vi "am_modul.vi"() -> ()   [LabVIEW 2015]
uses:
  <vilib>/express/express shared/transition.llb/Dynamic To Waveform Array.vi
  <vilib>/express/express arith-compare/Formula/Block/exnFormulaBlock how many pts in the wave.vi
  <vilib>/express/express shared/ex_Modify Signal Name.vi
  <vilib>/express/express shared/transition.llb/Waveform Array To Dynamic.vi
  <vilib>/express/express arith-compare/Formula/XNode/ExpressFormulaBlockNode.xnode
panel:
  out "String":string
  out "error out":errorcluster
  in  "stop":bool
  out "Graph demod AM-signal":dynamicdata(graph)
  out "f_demod_Hz":u32
  out "K_mod":dbl
  out "Graph AM-signal":dynamicdata(graph)
  in  "A_carry_V":dbl(knob) scale=0.1..0.3
  in  "F_mod_Hz":u32(knob) scale=40.0..280.0
  in  "A_mod_V":dbl(knob) scale=0.0..0.28
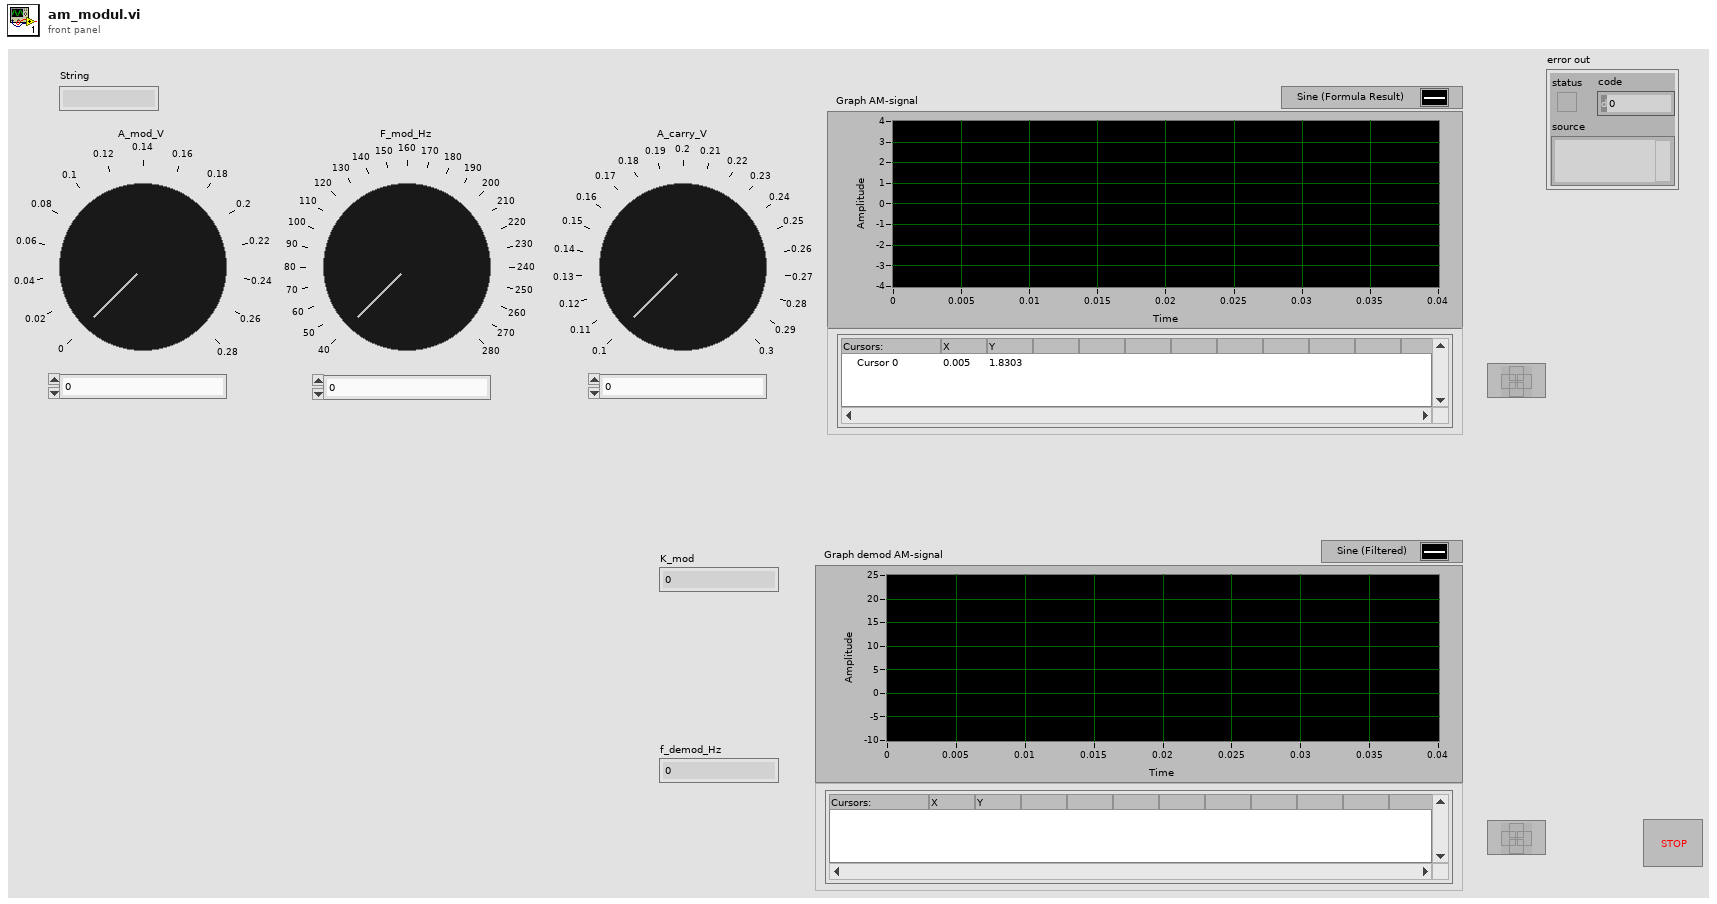
[diagram p1: front panel]
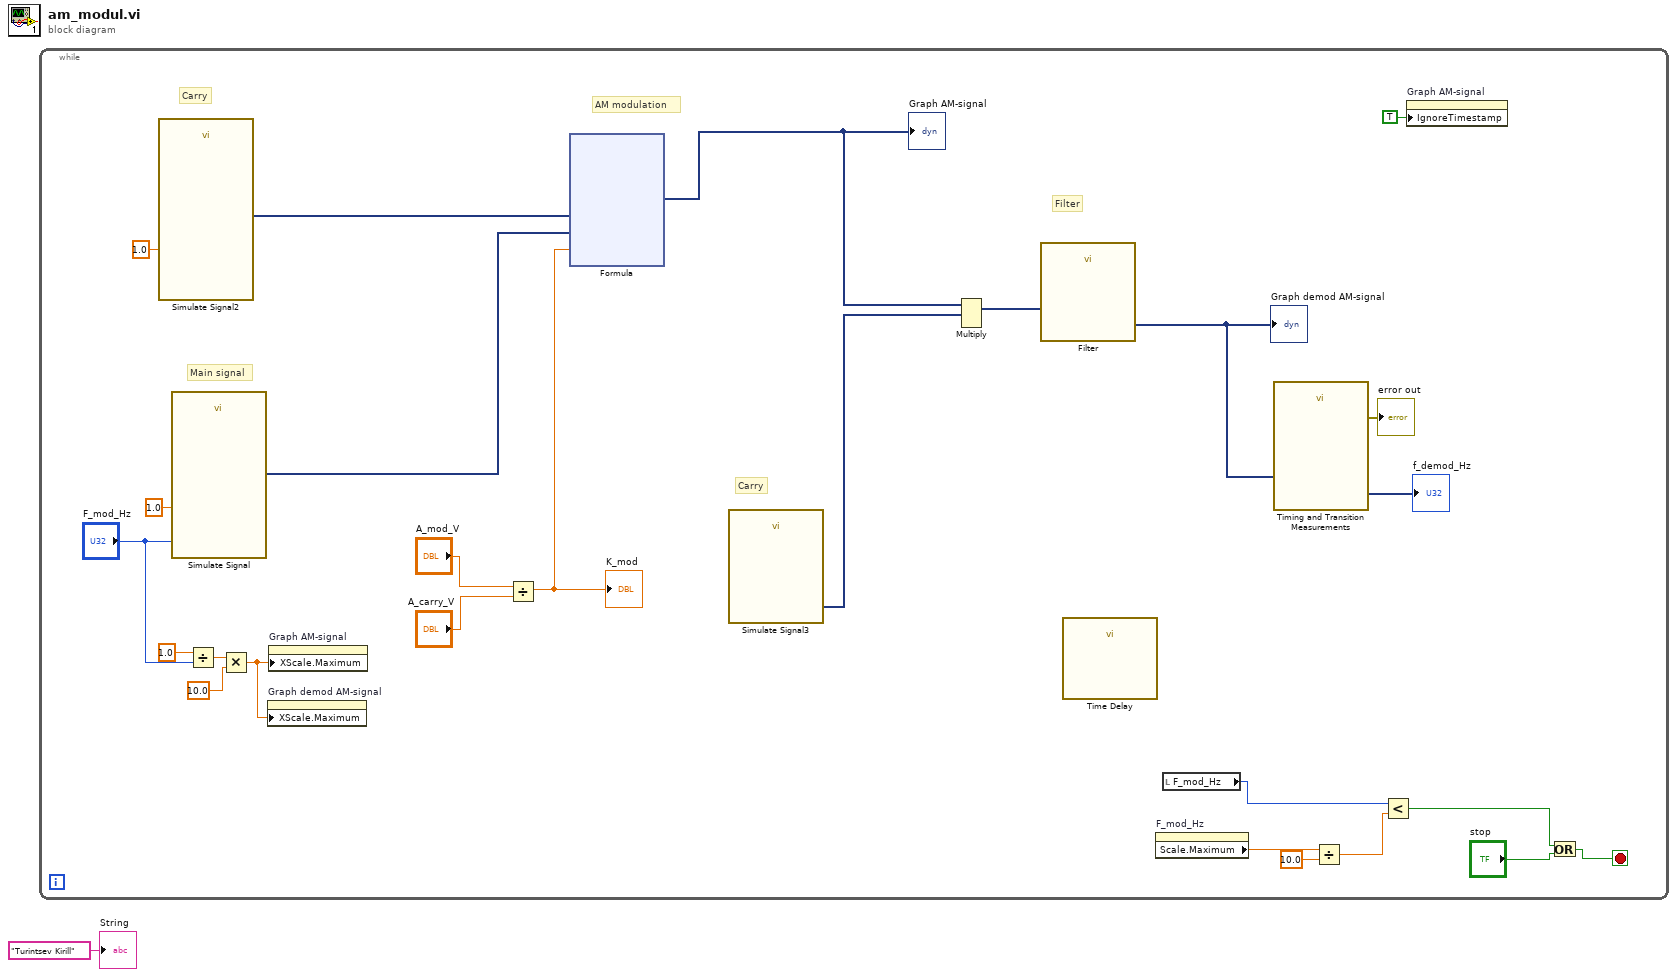
[diagram p0: block diagram]
diagram:
  n1 = while {
    stop <- w4 stop-if-true
    # "Filter"
    # "Carry"
    # "AM modulation"
    # "Main signal"
    # "Carry"
    n2 = call "Simulate Signal2"("Amplitude"=1.0) -> ("Sine"=w21:dynamicdata)  [unwired: 13 in, 1 out]
    n3 = call "Simulate Signal"("Frequency"="F_mod_Hz", "Amplitude"=1.0) -> ("Sine"=w22:dynamicdata)  [unwired: 12 in, 1 out]
    n4 = Divide(x=1.0, y="F_mod_Hz") -> (x/y=w12:dbl)
    n5 = Multiply(x=w12, y=10.0) -> (x*y=w10:dbl)
    n6 = property on="Graph demod AM-signal" class="WFGraph (strict)"("XScale.Maximum"=w10) -> ()  [unwired: 2 in, 2 out]
    n7 = property on="Graph AM-signal" class="WFGraph (strict)"("XScale.Maximum"=w10) -> ()  [unwired: 2 in, 2 out]
    n8 = Divide(x="A_mod_V", y="A_carry_V") -> (x/y=w20:dbl)
    "K_mod" <- w20
    n9 = xnode "Formula"("X2"=w21, "X1"=w22, "X3"=w20) -> ("Result"=w18:dynamicdata)  [unwired: 1 in, 1 out]
    "Graph AM-signal" <- w18
    n10 = call "Simulate Signal3"() -> ("Sine"=w19:dynamicdata)  [unwired: 14 in, 1 out]
    n11 = Multiply(1:w19, 2:w18) -> (0:w17:dynamicdata)  [unwired: 1 in, 1 out]
    n12 = call "Filter"("Signal"=w17) -> ("Filtered Signal"=w16:dynamicdata)  [unwired: 9 in, 1 out]
    "Graph demod AM-signal" <- w16
    n13 = call "Time Delay"() -> ()  [unwired: 11 in, 1 out]
    n14 = property on="F_mod_Hz" class="Knob (strict)"() -> ("Scale.Maximum"=w8:dbl)  [unwired: 2 in, 2 out]
    n15 = local read "F_mod_Hz"() -> (w6:u32)
    n16 = call "Timing and Transition Measurements"("Signals"=w16) -> ("error out"=→"error out":errorcluster, "Frequency"=→"f_demod_Hz":dynamicdata)  [unwired: 9 in]
    n17 = Divide(x=w8, y=10.0) -> (x/y=w5:dbl)
    n18 = Less?(x=w6, y=w5) -> (x < y?=w2:bool)
    n19 = property on="Graph AM-signal" class="WFGraph (strict)"("IgnoreTimestamp"=TRUE ("Ignore Timestamp")) -> ()  [unwired: 2 in, 2 out]
    n20 = Or(x=w2, y="stop") -> (x .or. y?=w4:bool)
  }
  "String" <- "Turintsev Kirill" ("String")
